vi "Add.vi"() -> ()   [LabVIEW 2012]
panel:
  in  "Numeric":dbl
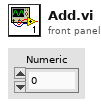
[diagram p1: front panel]
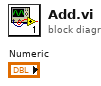
[diagram p0: block diagram]
diagram:
